vi "Scale_Factor.vi"(8 "Analogue In":dbl[][](array[numeric])) -> (0 "Analogue Out":dbl[][](array[numeric]))   [LabVIEW 2011]
uses:
  Globals/Meas_global.vi
  <vilib>/Utility/file.llb/Read From Spreadsheet File (string).vi
panel:
  out "Array":dbl[](array[numeric])
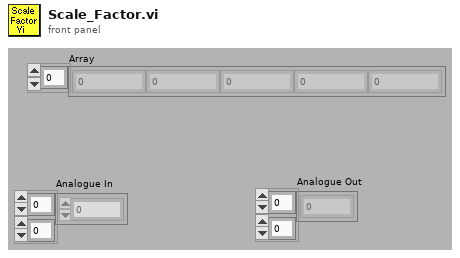
[diagram p1: front panel]
types:
  T1 = typedef "Analysis_info_cluster.ctl" = cluster{"Colour":u32, "Inst type":T2, "Inst name":string, "Symbol":string, "Code name":string, "Extra Info":string, "Inst Array":T3, "Index":i32, "Voltage Index":i32, "Extra Titles":string[], "Extra Values":string[], "Eng Values":dbl[], "Time (ms)":dbl[], "Voltage":dbl[], "U":dbl, "u^2":dbl, "u^3":dbl, "u^4":dbl, "Skew_u":dbl, "Kurt_u":dbl, "Sd Error in Mean":dbl, "% u'/U":dbl, "X":dbl, "Y":dbl, "Z":dbl, "Spectra":T4, "Autocorrelation":T4, "Timescale integral to 25%":dbl, "Sd Error in Variance":dbl, "Calib File":path, "Calib Constants":dbl[], "Histogram":T4, "Output Position":bool, "Full Stats":bool, "Weighting":dbl[]}
  T2 = typedef "Inst_type.ctl" = enum16{"Propeller anemometer", "Raw voltage", "Pressure Transducer", "Pitot-static tube", "Preston tube", "Hot wire", "Cross wire 1", "Cross wire 2", "Generic Linear", "Generic Polynomial", "Generic BackPoly", "Fast FID", "Thermocouple", "Cold wire", "Pulsed Wire", "LDA Vel", "LDA Tran time", "LDA Arr time"}
  T3 = typedef "Instrument_Array.ctl" = enum16{"PWA", "LDA", "Analogue"}
  T4 = typedef "XY_Plot_Cluster.ctl" = cluster{"First Name":string, "Second Name":string, "X axis name":string, "Y axis name":string, "X array":dbl[], "Y array":dbl[]}
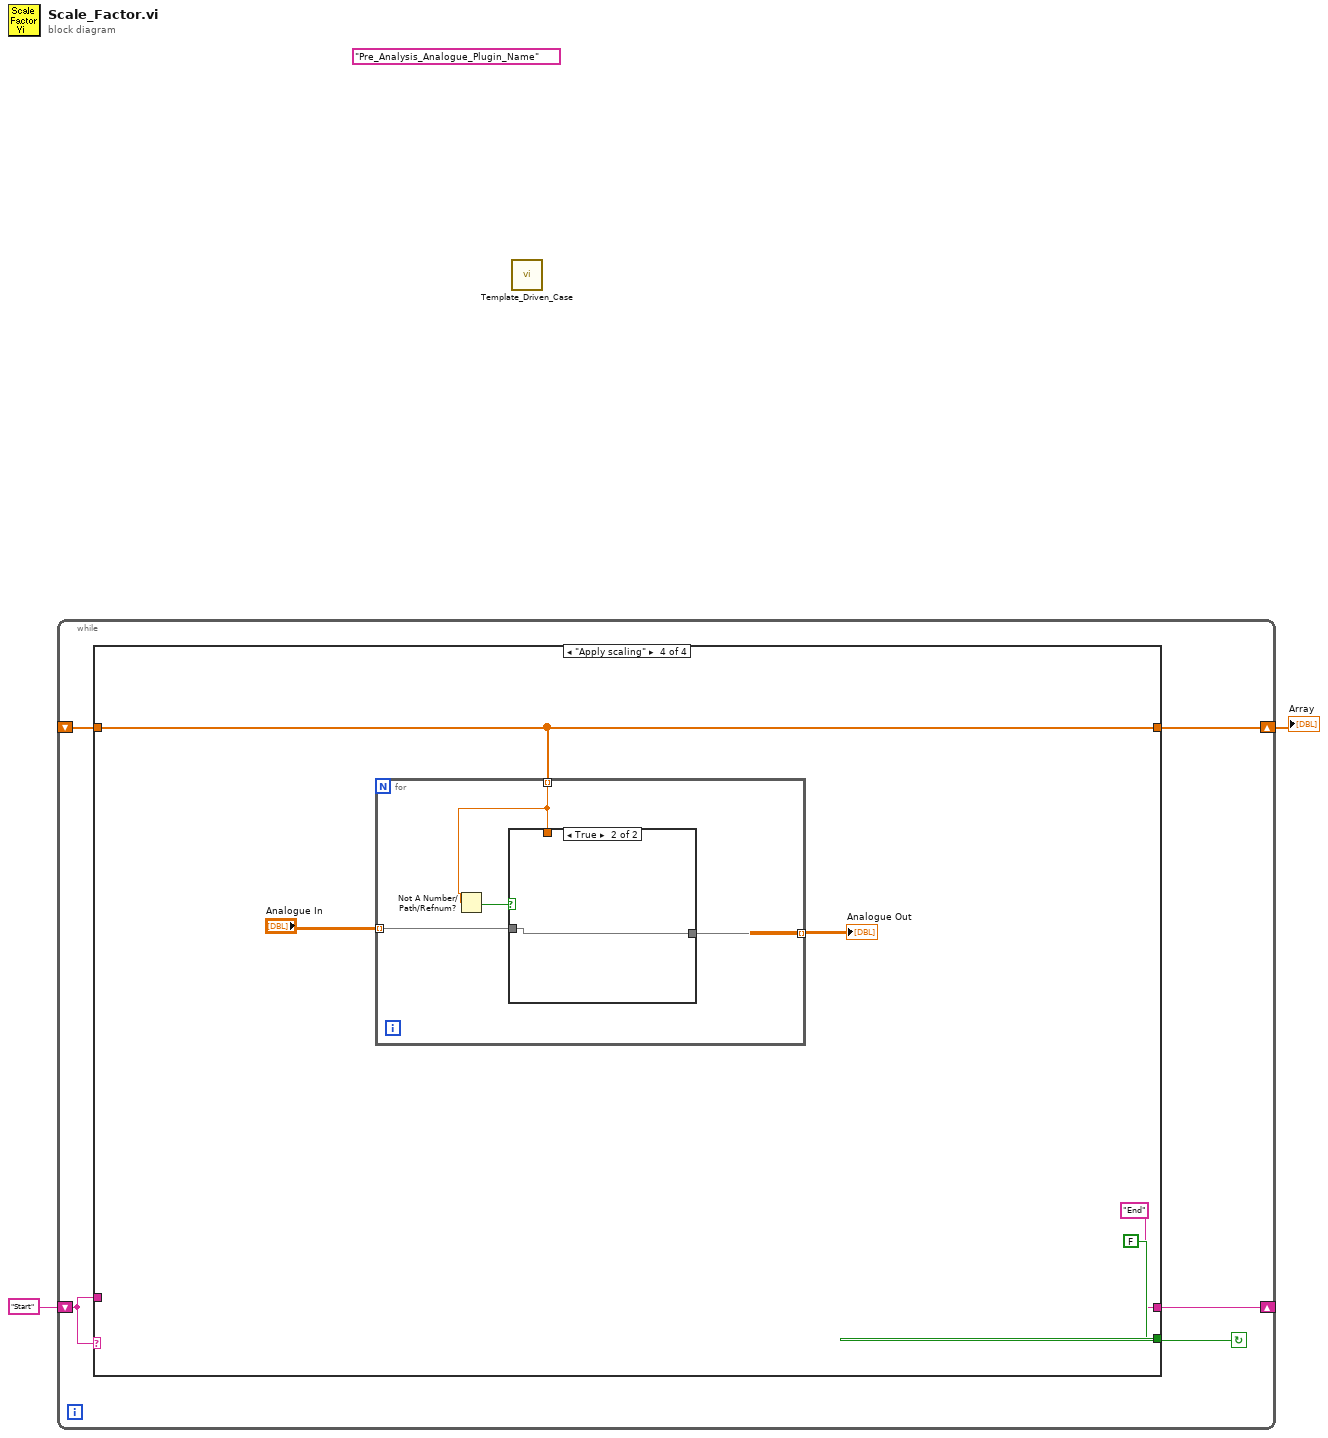
[diagram p0: block diagram]
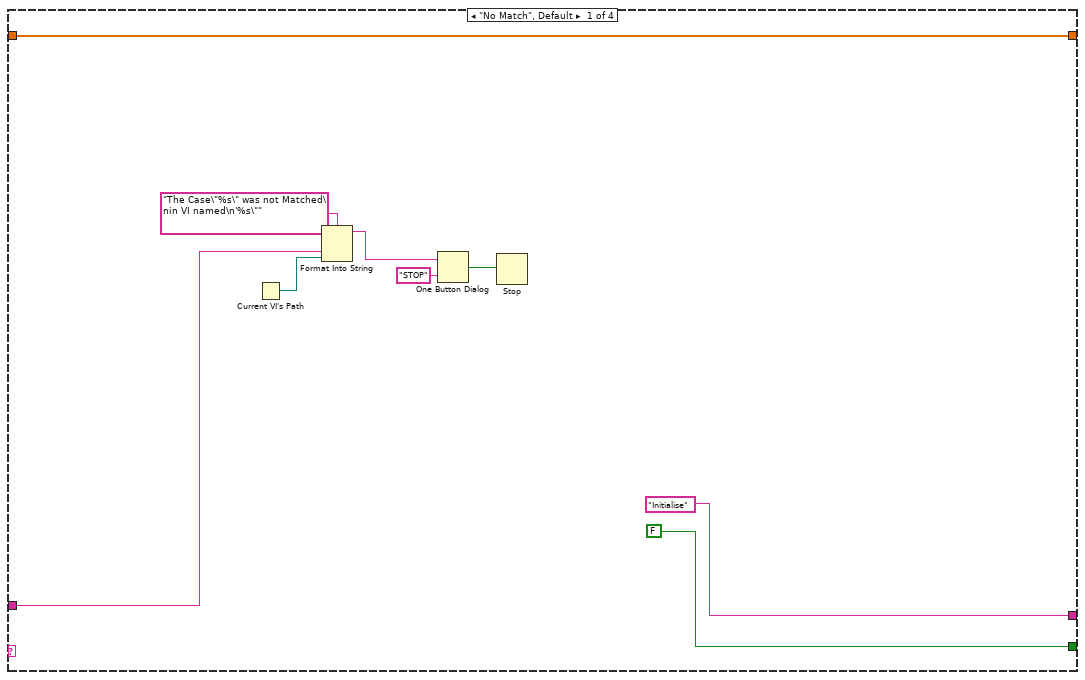
[diagram p2: hidden frame]
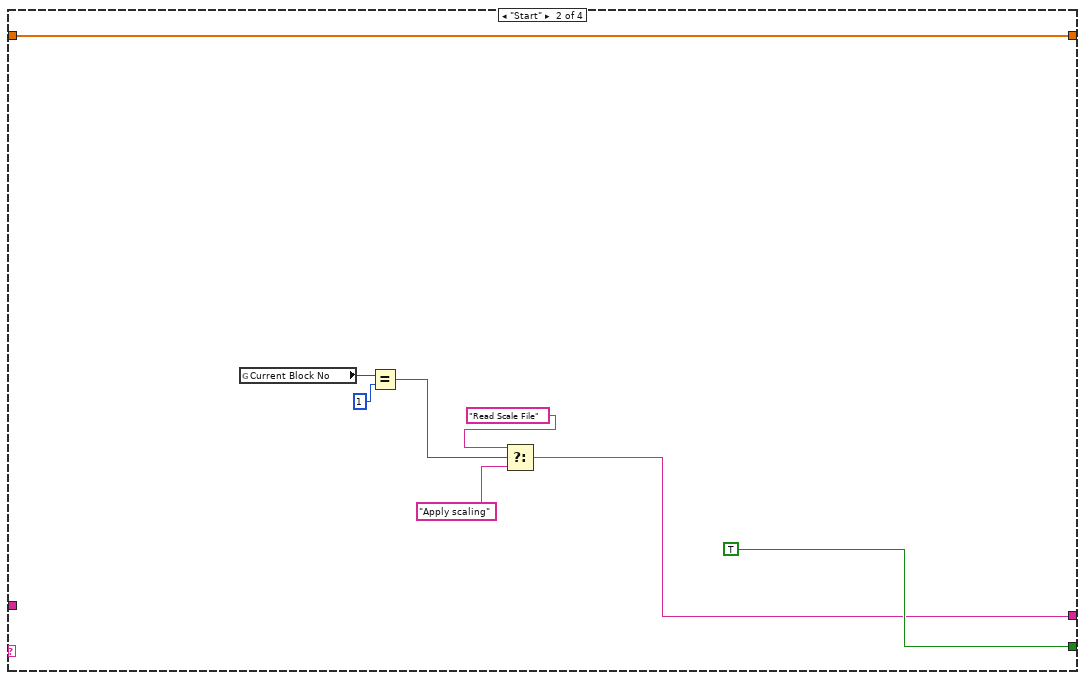
[diagram p3: hidden frame]
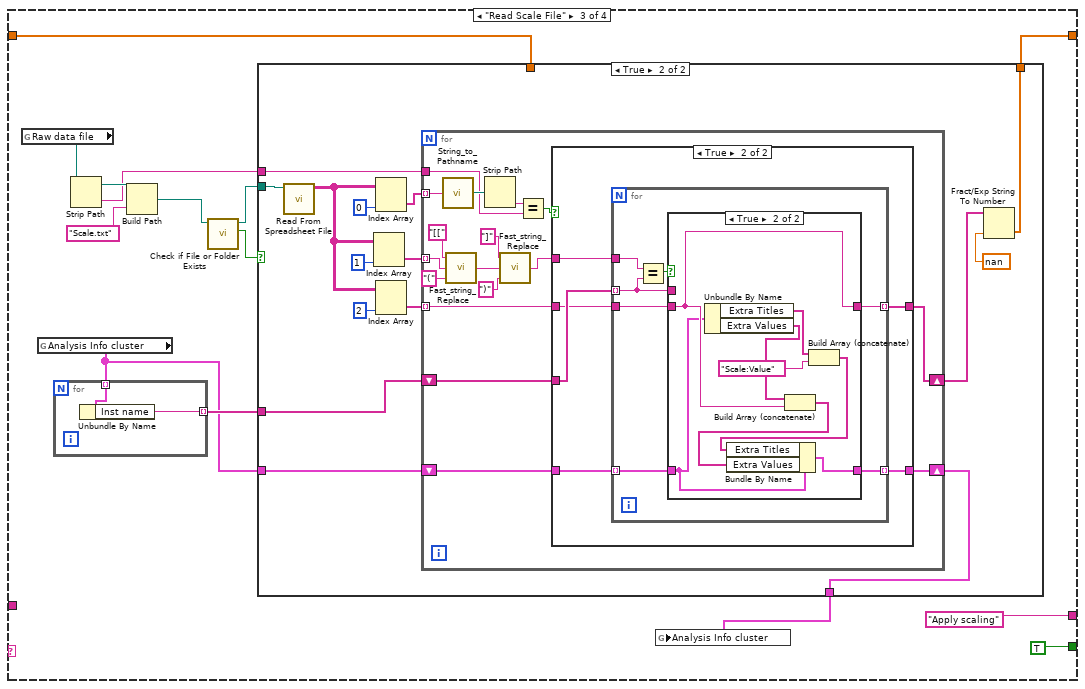
[diagram p4: hidden frame]
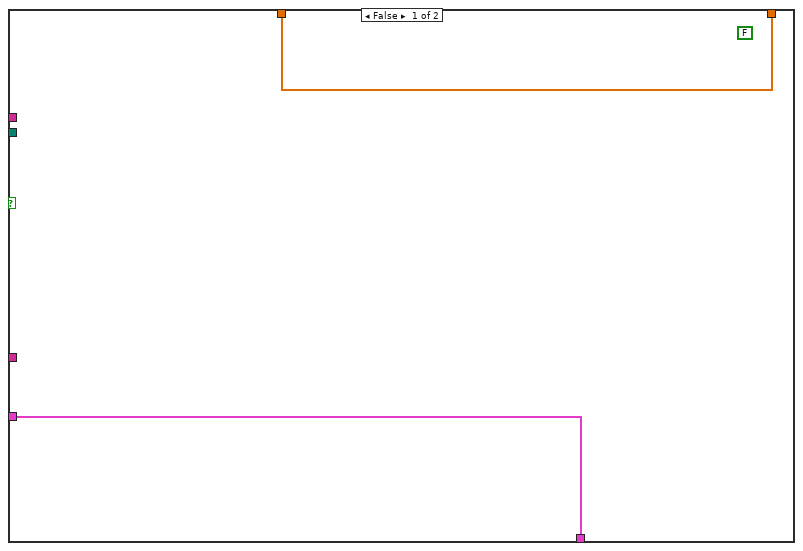
[diagram p5: hidden frame]
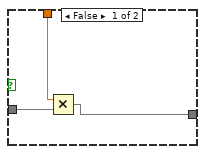
[diagram p8: hidden frame]
diagram:
  (unwired) "Pre_Analysis_Analogue_Plugin_Name"
  n1 = while {
    shift-left: "Start" -> [w5]
    shift-right: [w6] -> _
    shift-right: [w4] -> w1
    shift-left: _ -> [w3]
    stop <- w7 continue-if-true
    n2 = case shown="\"Apply scaling\"" w5 {
      tunnel: [FALSE TRUE TRUE FALSE] -> w7
      tunnel: ["Initialise" w21 "Apply scaling" "End" ("f")] -> w6
      tunnel: w5 -> [w11 _ _ _]
      tunnel: [w8 w20 w26 w102] -> w4
      tunnel: w3 -> [w8 w20 w29 w102]
      frame "No Match", Default {
        n3 = Current VI's Path() -> (path=w10:path)
        n4 = Format Into String(format string="The Case\"%s\" was not Matched\nin VI named\n'%s\"" ("Format String"), w11, w10) -> (resulting string=w14:string)  [unwired: 2 in, 1 out]
        n5 = One Button Dialog(message=w14, button name ("OK")="STOP") -> (true=w12:bool)
        n6 = Stop(stop? (T)=w12) -> ()
      }
      frame "Start" {
        n7 = global read "Meas_global.vi" "Current Block No"() -> (w19:i32)
        n8 = Equal?(x=w19, y=1) -> (x = y?=w17:bool)
        n9 = Select(t="Read Scale File", s=w17, f="Apply scaling") -> (s? t:f=w21:string)
      }
      frame "Read Scale File" {
        n10 = global read "Meas_global.vi" "Raw data file"() -> (w37:path)
        n11 = global read "Meas_global.vi" "Analysis Info cluster"() -> (w27:T1[])
        n12 = for {
          tunnel: w27 -> [w40] mode=indexing
          tunnel: [w39] -> w30 mode=indexing
          n13 = Unbundle By Name(w40) -> ("Inst name"=w39:string)
        }
        n14 = Strip Path(path=w37) -> (stripped path=w36:path, name=w31:string)
        n15 = Build Path(base path=w36, name or relative path="Scale.txt") -> (appended path=w34:path)
        n16 = call <vilib>:"Check if File or Folder Exists.vi"("path"=w34) -> ("file or folder exists?"=w32:bool, "dup path"=w33:path)  [unwired: 1 in, 8 out]
        n17 = case shown="True" w32 {
          tunnel: w33 -> [_ w57]
          tunnel: w31 -> [_ w55]
          tunnel: w30 -> [_ w54]
          tunnel: [w42 w46] -> w26
          tunnel: w29 -> [w42 _]
          tunnel: w27 -> [w41 w44]
          tunnel: [w41 w43] -> w25
          frame False {
            (unwired) FALSE
          }
          frame True {
            n18 = call-poly <vilib>:"Read From Spreadsheet File.vi"("file path (dialog if empty)"=w57) -> ("all rows"=w49:string[][])  [unwired: 3 in, 7 out]
            n19 = Index Array(array=w49, index (col)=1 ("disabled index (col)")) -> (element=w50:string[])  [unwired: 1 in]
            n20 = Index Array(array=w49, index (col)=0 ("disabled index (col)")) -> (element=w56:string[])  [unwired: 1 in]
            n21 = Index Array(array=w49, index (col)=2 ("disabled index (col)")) -> (element=w48:string[])  [unwired: 1 in]
            n22 = for {
              tunnel: w56 -> [w74] mode=indexing
              shift-right: [w68] -> w47
              shift-left: w54 -> [w69]
              tunnel: w55 -> [w71]
              tunnel: w50 -> [w66] mode=indexing
              tunnel: w48 -> [w67] mode=indexing
              shift-right: [w58] -> w43
              shift-left: w44 -> [w59]
              n23 = call "String_to_Pathname.vi"("Input String"=w74) -> ("path"=w73:path)
              n24 = call "Fast_string_Replace.vi"("Replace match with:"="(", "Input String"=w66, "regular expression"="[[") -> ("Output String"=w65:string)  [unwired: 2 out]
              n25 = Strip Path(path=w73) -> (name=w72:string)  [unwired: 1 out]
              n26 = call "Fast_string_Replace.vi"("Replace match with:"=")", "Input String"=w65, "regular expression"="]") -> ("Output String"=w64:string)  [unwired: 2 out]
              n27 = Equal?(x=w72, y=w71) -> (x = y?=w70:bool)
              n28 = case shown="True" w70 {
                tunnel: w69 -> [w76 w82]
                tunnel: [w76 w79] -> w68
                tunnel: w64 -> [_ w81]
                tunnel: w67 -> [_ w80]
                tunnel: w59 -> [w75 w78]
                tunnel: [w75 w77] -> w58
                frame False {
                }
                frame True {
                  n29 = for {
                    tunnel: w82 -> [w85] mode=indexing
                    tunnel: w81 -> [w89]
                    tunnel: w80 -> [w87]
                    tunnel: [w86] -> w79 mode=indexing
                    tunnel: w78 -> [w84] mode=indexing
                    tunnel: [w83] -> w77 mode=indexing
                    n30 = Equal?(x=w89, y=w85) -> (x = y?=w88:bool)
                    n31 = case shown="True" w88 {
                      tunnel: w87 -> [_ w97]
                      tunnel: [w91 w97] -> w86
                      tunnel: w85 -> [w91 _]
                      tunnel: w84 -> [w90 w96]
                      tunnel: [w90 w93] -> w83
                      frame False {
                      }
                      frame True {
                        n32 = Unbundle By Name(w96) -> ("Extra Titles"=w99:string[], "Extra Values"=w98:string[])
                        n33 = Build Array (concatenate)(w98, w97) -> (w94:string[])
                        n34 = Build Array (concatenate)(w99, "Scale:Value" ("string")) -> (w95:string[])
                        n35 = Bundle By Name(cluster=w96, "Extra Titles"=w95, "Extra Values"=w94) -> (w93:T1)
                      }
                    }
                  }
                }
              }
            }
            n36 = Fract/Exp String To Number(string=w47, default (0 dbl)=nan ("default (0 DBL)")) -> (number=w46:dbl[])  [unwired: 3 out]
          }
        }
        n37 = global write "Meas_global.vi" "Analysis Info cluster"(w25) -> ()
      }
      frame "Apply scaling" {
        n38 = for {
          tunnel: w102 -> [w105] mode=indexing
          tunnel: "Analogue In" -> [w108] mode=indexing
          tunnel: [w107] -> w103 mode=indexing
          n39 = Not A Number/Path/Refnum?(number/path/refnum=w105) -> (NaN/Path/Refnum?=w106:bool)
          n40 = case shown="True" w106 {
            tunnel: w105 -> [w111 _]
            tunnel: w108 -> [w110 w112]
            tunnel: [w109 w112] -> w107
            frame False {
              n41 = Multiply(x=w111, y=w110) -> (x*y=w109:dbl[])
            }
            frame True {
            }
          }
        }
        "Analogue Out" <- w103
      }
    }
  }
  "Array" <- w1
  n42 = call "Template_Driven_Case.vi"() -> ()  [unwired: 1 out]
